vi "ip_change_sql.vi"() -> ()   [LabVIEW 2022 SP3]
panel:
  out "error out":errorcluster
  in  "cancel":bool
  in  "new_IP":string
  out "status":string
  in  "ok":bool
  in  "intrface_name":string(combo)
  in  "error in (no error)":errorcluster
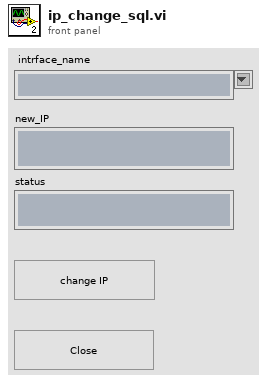
[diagram p1: front panel]
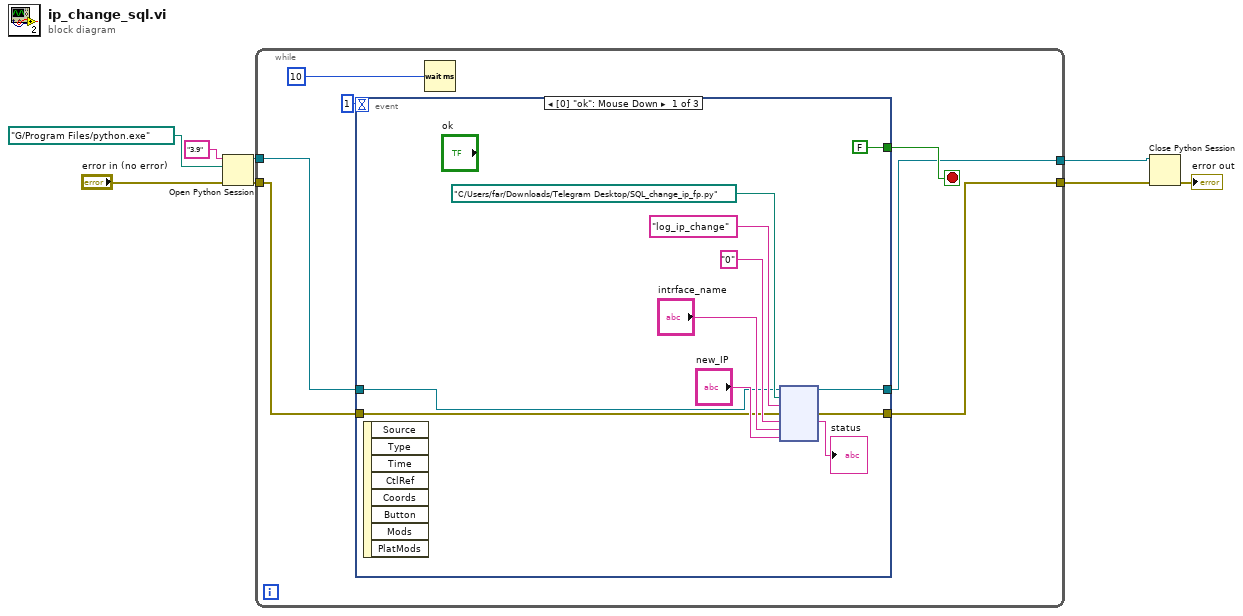
[diagram p0: block diagram]
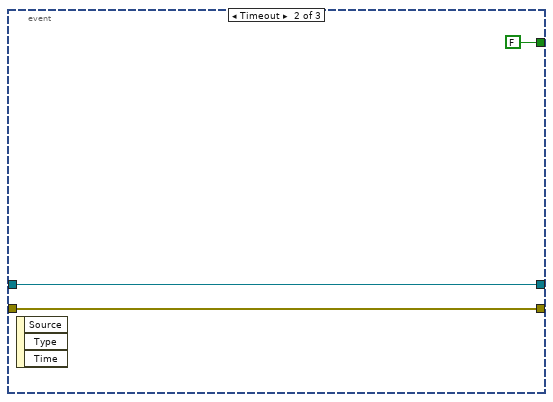
[diagram p2: hidden frame]
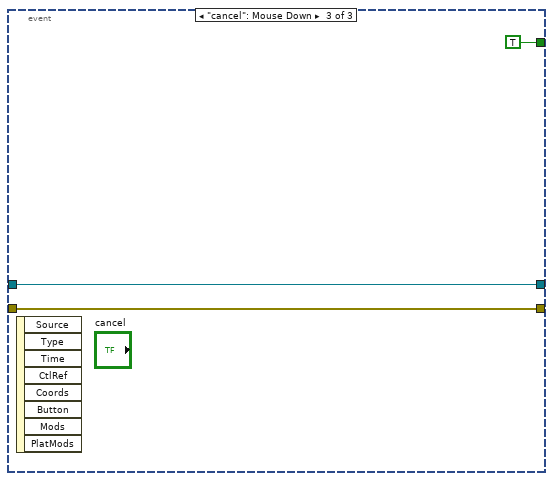
[diagram p3: hidden frame]
diagram:
  n1 = Open Python Session(python version="3.9" ("Python version"), python path=path "G:/Program Files/python.exe" ("Python path"), 3:"error in (no error)") -> (session out=w5:refnum<k35>, error out=w4:errorcluster)
  n2 = while {
    tunnel: w5 -> [w15]
    tunnel: w4 -> [w10]
    tunnel: [w14] -> w3
    tunnel: [w9] -> w1
    stop <- w11 stop-if-true
    n3 = event shown="[0] \"ok\": Mouse Down" {
      selector: _ -> [_ _ _]
      dyn-events: _ -> [_ _ _]
      timeout: 1 -> [_ _ _]
      tunnel: w15 -> [w19 w29 w32]
      tunnel: w10 -> [w18 w28 w31]
      tunnel: [w17 w29 w32] -> w9
      tunnel: [w16 w28 w31] -> w14
      tunnel: [FALSE ("cancel") FALSE ("cancel") TRUE ("cancel")] -> w11
      event "ok": Mouse Down {
        n4 = event-data() -> ()  [unwired: 1 in, 8 out]
        n5 = node(w19, path "C:/Users/far/Downloads/Telegram Desktop/SQL_change_ip_fp.py" ("module path"), "log_ip_change" ("function name"), w18, "0", "intrface_name", "new_IP") -> (w17:refnum<k35>, w16:errorcluster, →"status":string)  [unwired: 2 in, 2 out]
      }
      event Timeout {
        n6 = event-data() -> ()  [unwired: 1 in, 3 out]
      }
      event "cancel": Mouse Down {
        n7 = event-data() -> ()  [unwired: 1 in, 8 out]
      }
    }
    n8 = Wait (ms)(milliseconds to wait=u32 10) -> ()  [unwired: 1 out]
  }
  n9 = Close Python Session(session in=w1, error in=w3) -> (11:→"error out":errorcluster)
